vi "RF Waveform Builder.vi"() -> ()   [LabVIEW 2018]
uses:
  <vilib>/Analysis/NI_AALBase.lvlib
panel:
  in  "Delay(s)":dbl
  in  "Duration(s)":dbl
  in  "Amplitdue":dbl
  in  "Sample Rate (Sa/S)":dbl
  in  "Frequency(Hz)":dbl
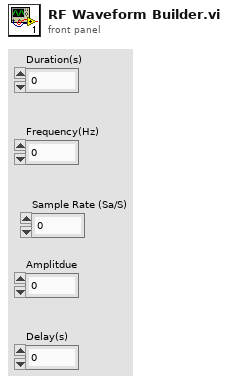
[diagram p1: front panel]
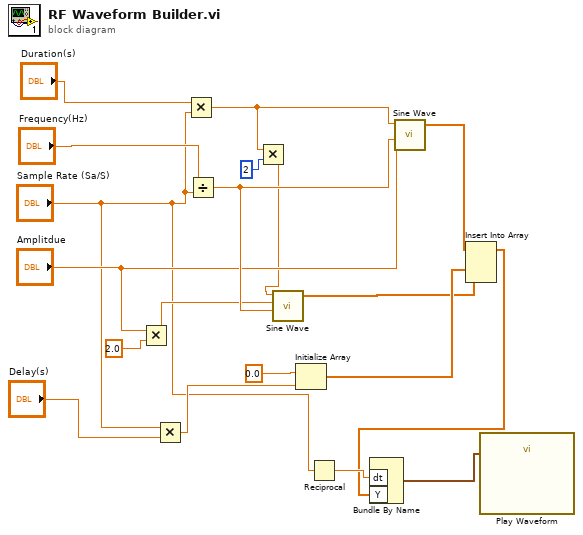
[diagram p0: block diagram]
diagram:
  n1 = Multiply(x="Amplitdue", y=2.0) -> (x*y=w16:dbl)
  n2 = Multiply(x="Sample Rate (Sa/S)", y="Delay(s)") -> (x*y=w11:dbl)
  n3 = Multiply(x="Duration(s)", y="Sample Rate (Sa/S)") -> (x*y=w3:dbl)
  n4 = Divide(x="Frequency(Hz)", y="Sample Rate (Sa/S)") -> (x/y=w18:dbl)
  n5 = Multiply(x=w3, y=2) -> (x*y=w1:dbl)
  n6 = call <vilib>:"Sine Wave.vi"("samples"=w1, "amplitude"=w16, "frequency"=w18) -> ("sine wave"=w8:dbl[])  [unwired: 2 in, 2 out]
  n7 = Initialize Array(0.0, w11) -> (w9:dbl[])
  n8 = Reciprocal(x="Sample Rate (Sa/S)") -> (1/x=w7:dbl)
  n9 = call <vilib>:"Sine Wave.vi"("samples"=w3, "amplitude"="Amplitdue", "frequency"=w18) -> ("sine wave"=w15:dbl[])  [unwired: 2 in, 2 out]
  n10 = Insert Into Array(array=w15, new element #1=w9, new element #2=w8) -> (w5:dbl[])  [unwired: 1 in]
  n11 = Bundle By Name("dt"=w7, "Y"=w5) -> (w4:waveform(dbl))  [unwired: 1 in]
  n12 = call "Play Waveform"("Data"=w4) -> ()  [unwired: 18 in, 1 out]
